vi "ChartsAndGraphs.vi"() -> ()   [LabVIEW 2011]
uses:
  <vilib>/ptbypt/NI_PtbyPt.lvlib
panel:
  in  "stop":bool
  in  "time step (s)":dbl=0.25
  in  "phase":dbl format="%0.2f"
  in  "frequency":dbl=0.5 format="%0.2f"
  in  "amplitude":dbl=1.0 format="%0.2f"
  out "XY Graph":cluster{dbl[], dbl[]}(graph)
  out "Waveform Graph":waveform(dbl)(graph)
  out "Waveform Chart":dbl(graph)
  # "Sine wave"
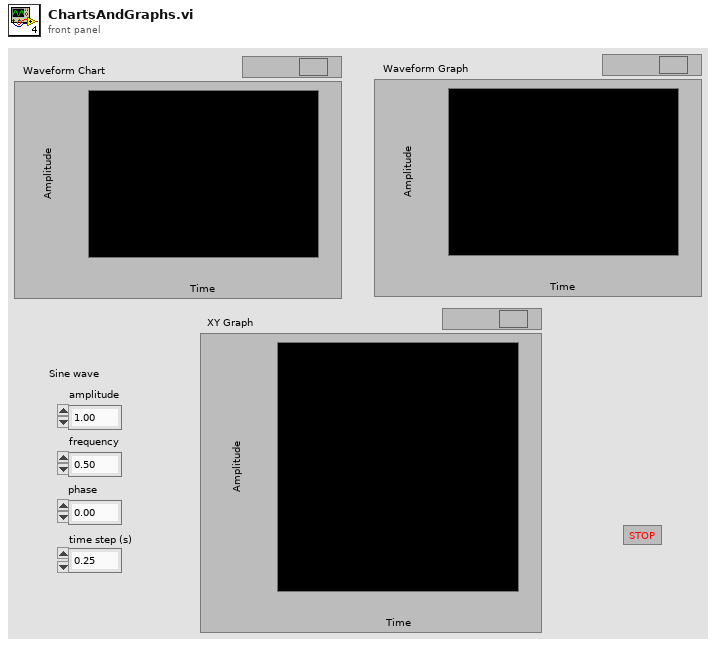
[diagram p1: front panel]
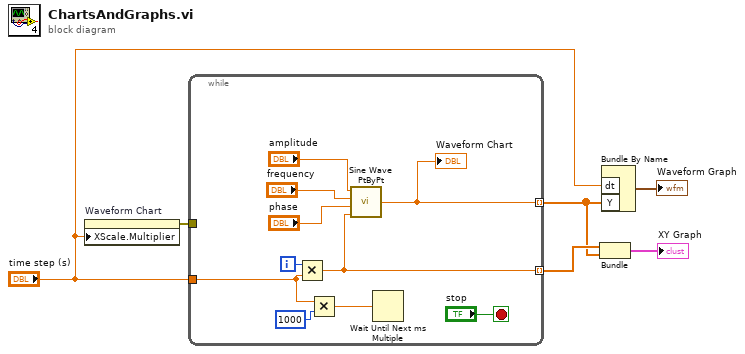
[diagram p0: block diagram]
diagram:
  n1 = property on="Waveform Chart" class="WFChart (strict)"("XScale.Multiplier"="time step (s)") -> (error out=w6:errorcluster)  [unwired: 2 in, 1 out]
  n2 = while {
    tunnel: [w13] -> w3 mode=indexing
    tunnel: [w8] -> w5 mode=indexing
    tunnel: "time step (s)" -> [w11]
    tunnel: w6 -> [_]
    i -> [w12]
    stop <- "stop" stop-if-true
    n3 = Multiply(x=w12, y=w11) -> (x*y=w8:dbl)
    n4 = Multiply(x=w11, y=u32 1000 ("millisecond multiple")) -> (x*y=w9:dbl)
    n5 = call <vilib>:"Sine Wave PtByPt.vi"("time"=w8, "phase"="phase", "frequency"="frequency", "amplitude"="amplitude") -> ("sine wave"=w13:dbl)
    "Waveform Chart" <- w13
    n6 = Wait Until Next ms Multiple(millisecond multiple=w9) -> ()  [unwired: 1 out]
  }
  n7 = Bundle(w5, w3) -> (→"XY Graph":cluster{dbl[], dbl[]})  [unwired: 1 in]
  n8 = Bundle By Name("dt"="time step (s)", "Y"=w3) -> (→"Waveform Graph":waveform(dbl))  [unwired: 1 in]
